vi "test_read-nmea-data2.vi"() -> ()   [LabVIEW 2019] (continued)
,86,148,25,33,59,218,30,1*43\n\t\n15:09:04.70\tF9P\t$GBGSV,2,1,05,08,,,28,10,,,07,11,51,130,29,14,86,148,31,3*7F\n\t\n15:09:04.72\tF9P\t$GBGSV,2,2,05,33,59,218,,3*46\n\t\n15:09:04.74\tF9P\t$GNGLL,3723.60830,N,12656.91746,E,060906.00,A,A*7D\n\t\n15:09:04.76\tF9P\t\t\n15:09:04.78\tF9P\t\t\n15:09:04.80\tF9P\t\t\n15:09:04.82\tF9P\t\t\n15:09:04.84\tF9P\t\t\n15:09:04.86\tF9P\t\t\n15:09:04.88\tF9P\t\t\n15:09:04.90\tF9P\t\t\n15:09:04.92\tF9P\t\t\n15:09:04.94\tF9P\t\t\n15:09:04.96\tF9P\t\t\n15:09:04.98\tF9P\t\t\n15:09:05.00\tF9P\t\t\n15:09:05.02\tF9P\t\t\n15:09:05.04\tF9P\t\t\n15:09:05.06\tF9P\t\t\n15:09:05.08\tF9P\t\t\n15:09:05.10\tF9P\t\t\n15:09:05.12\tF9P\t\t\n15:09:05.14\tF9P\t\t\n15:09:05.16\tF9P\t\t\n15:09:05.18\tF9P\t\t\n15:09:05.20\tF9P\t\t\n15:09:05.22\tF9P\t\t\n15:09:05.24\tF9P\t\t\n15:09:05.26\tF9P\t$GNRMC,060907.00,A,3723.60831,N,12656.91695,E,1.891,293.46,250720,,,A,V*06\n\t\n15:09:05.28\tF9P\t$GNVTG,293.46,T,,M,1.891,N,3.502,K,A*2C\n\t\n15:09:05.30\tF9P\t$GNGGA,060907.00,3723.60831,N,12656.91695,E,1,12,0.72,59.0,M,18.5,M,,*71\n\t\n15:09:05.32\tF9P\t$GNGSA,A,3,12,06,19,05,17,09,04,02,,,,,1.25,0.72,1.02,1*00\n\t\n15:09:05.34\tF9P\t$GNGSA,A,3,70,85,71,84,,,,,,,,,1.25,0.72,1.02,2*02\n\t\n15:09:05.36\tF9P\t$GNGSA,A,3,36,19,11,04,09,12,,,,,,,1.25,0.72,1.02,3*00\n\t\n15:09:05.38\tF9P\t$GNGSA,A,3,14,11,33,,,,,,,,,,1.25,0.72,1.02,4*01\n\t\n15:09:05.40\tF9P\t$GPGSV,3,1,09,02,54,318,26,04,19,044,26,05,36,246,25,06,65,046,28,1*60\n\t\n15:09:05.42\tF9P\t$GPGSV,3,2,09,09,45,076,35,12,24,278,29,17,35,153,24,19,54,156,24,1*6C\n\t\n15:09:05.44\tF9P\t$GPGSV,3,3,09,25,12,308,,1*52\n\t\n15:09:05.46\tF9P\t$GPGSV,3,1,09,02,54,318,,04,19,044,20,05,36,246,17,06,65,046,23,6*6F\n\t\n15:09:05.48\tF9P\t$GPGSV,3,2,09,09,45,076,20,12,24,278,22,17,35,153,,19,54,156,,6*64\n\t\n15:09:05.50\tF9P\t$GPGSV,3,3,09,25,12,308,,6*55\n\t\n15:09:05.52\tF9P\t$GLGSV,2,1,08,69,13,031,,70,73,042,21,71,50,204,27,72,03,209,,1*77\n\t\n15:09:05.54\tF9P\t$GLGSV,2,2,08,77,01,327,,84,21,121,10,85,70,063,25,86,35,329,,1*73\n\t\n15:09:05.56\tF9P\t$GLGSV,2,1,08,69,13,031,,70,73,042,,71,50,204,22,72,03,209,,3*73\n\t\n15:09:05.58\tF9P\t$GLGSV,2,2,08,77,01,327,,84,21,121,18,85,70,063,23,86,35,329,,3*7F\n\t\n15:09:05.60\tF9P\t$GAGSV,2,1,08,02,09,298,10,04,65,120,25,09,30,193,24,11,70,356,30,7*71\n\t\n15:09:05.62\tF9P\t$GAGSV,2,2,08,12,41,101,25,19,27,046,24,25,10,250,,36,25,307,20,7*76\n\t\n15:09:05.64\tF9P\t$GAGSV,2,1,08,02,09,298,,04,65,120,33,09,30,193,,11,70,356,27,2*72\n\t\n15:09:05.66\tF9P\t$GAGSV,2,2,08,12,41,101,20,19,27,046,19,25,10,250,,36,25,307,14,2*7F\n\t\n15:09:05.68\tF9P\t$GBGSV,1,1,03,11,51,130,26,14,86,148,25,33,59,218,29,1*4A\n\t\n15:09:05.70\tF9P\t$GBGSV,2,1,05,08,,,29,10,,,07,11,51,130,27,14,86,148,31,3*70\n\t\n15:09:05.72\tF9P\t$GBGSV,2,2,05,33,59,218,,3*46\n\t\n15:09:05.74\tF9P\t$GNGLL,3723.60831,N,12656.91695,E,060907.00,A,A*72\n\t\n15:09:05.76\tF9P\t\t\n15:09:05.78\tF9P\t\t\n15:09:05.80\tF9P\t\t\n15:09:05.82\tF9P\t\t\n15:09:05.84\tF9P\t\t\n15:09:05.86\tF9P\t\t\n15:09:05.88\tF9P\t\t\n15:09:05.90\tF9P\t\t\n15:09:05.92\tF9P\t\t\n15:09:05.94\tF9P\t\t\n15:09:05.96\tF9P\t\t\n15:09:05.98\tF9P\t\t\n15:09:06.00\tF9P\t\t\n15:09:06.02\tF9P\t\t\n15:09:06.04\tF9P\t\t\n15:09:06.06\tF9P\t\t\n15:09:06.08\tF9P\t\t\n15:09:06.10\tF9P\t\t\n15:09:06.12\tF9P\t\t\n15:09:06.14\tF9P\t\t\n15:09:06.16\tF9P\t\t\n15:09:06.18\tF9P\t\t\n15:09:06.20\tF9P\t\t\n15:09:06.22\tF9P\t\t\n15:09:06.24\tF9P\t\t\n15:09:06.26\tF9P\t$GNRMC,060908.00,A,3723.60810,N,12656.91634,E,2.095,270.86,250720,,,A,V*0F\n\t\n15:09:06.28\tF9P\t$GNVTG,270.86,T,,M,2.095,N,3.879,K,A*23\n\t\n15:09:06.30\tF9P\t$GNGGA,060908.00,3723.60810,N,12656.91634,E,1,12,0.68,59.0,M,18.5,M,,*7D\n\t\n15:09:06.32\tF9P\t$GNGSA,A,3,12,06,19,05,17,09,04,02,,,,,1.22,0.68,1.01,1*0F\n\t\n15:09:06.34\tF9P\t$GNGSA,A,3,70,85,71,84,,,,,,,,,1.22,0.68,1.01,2*0D\n\t\n15:09:06.36\tF9P\t$GNGSA,A,3,36,19,11,04,09,12,,,,,,,1.22,0.68,1.01,3*0F\n\t\n15:09:06.38\tF9P\t$GNGSA,A,3,14,11,33,,,,,,,,,,1.22,0.68,1.01,4*0E\n\t\n15:09:06.40\tF9P\t$GPGSV,3,1,09,02,54,318,25,04,19,044,26,05,36,246,28,06,65,046,29,1*6F\n\t\n15:09:06.42\tF9P\t$GPGSV,3,2,09,09,45,076,33,12,24,278,28,17,35,153,26,19,54,156,26,1*6B\n\t\n15:09:06.44\tF9P\t$GPGSV,3,3,09,25,12,308,,1*52\n\t\n15:09:06.46\tF9P\t$GPGSV,3,1,09,02,54,318,,04,19,044,20,05,36,246,19,06,65,046,25,6*67\n\t\n15:09:06.48\tF9P\t$GPGSV,3,2,09,09,45,076,21,12,24,278,21,17,35,153,,19,54,156,,6*66\n\t\n15:09:06.50\tF9P\t$GPGSV,3,3,09,25,12,308,,6*55\n\t\n15:09:06.52\tF9P\t$GLGSV,2,1,08,69,13,031,,70,73,042,18,71,50,204,27,72,03,209,,1*7D\n\t\n15:09:06.54\tF9P\t$GLGSV,2,2,08,77,01,327,,84,21,121,07,85,70,063,24,86,35,329,,1*74\n\t\n15:09:06.56\tF9P\t$GLGSV,2,1,08,69,13,031,21,70,73,042,,71,50,204,21,72,03,209,,3*73\n\t\n15:09:06.58\tF9P\t$GLGSV,2,2,08,77,01,327,,84,21,121,19,85,70,063,25,86,35,329,,3*78\n\t\n15:09:06.60\tF9P\t$GAGSV,2,1,08,02,09,298,07,04,65,120,24,09,30,193,24,11,70,356,24,7*73\n\t\n15:09:06.62\tF9P\t$GAGSV,2,2,08,12,41,101,23,19,27,046,20,25,10,250,,36,25,307,19,7*7E\n\t\n15:09:06.64\tF9P\t$GAGSV,2,1,08,02,09,298,,04,65,120,33,09,30,193,22,11,70,356,26,2*73\n\t\n15:09:06.66\tF9P\t$GAGSV,2,2,08,12,41,101,18,19,27,046,18,25,10,250,,36,25,307,20,2*72\n\t\n15:09:06.68\tF9P\t$GBGSV,1,1,03,11,51,130,25,14,86,148,30,33,59,218,29,1*4D\n\t\n15:09:06.70\tF9P\t$GBGSV,2,1,05,08,,,30,10,,,08,11,51,130,26,14,86,148,27,3*71\n\t\n15:09:06.72\tF9P\t$GBGSV,2,2,05,33,59,218,,3*46\n\t\n15:09:06.74\tF9P\t$GNGLL,3723.60810,N,12656.91634,E,060908.00,A,A*75\n\t\n15:09:06.76\tF9P\t\t\n15:09:06.78\tF9P\t\t\n15:09:06.80\tF9P\t\t\n15:09:06.82\tF9P\t\t\n15:09:06.84\tF9P\t\t\n15:09:06.86\tF9P\t\t\n15:09:06.88\tF9P\t\t\n15:09:06.90\tF9P\t\t\n15:09:06.92\tF9P\t\t\n15:09:06.94\tF9P\t\t\n15:09:06.96\tF9P\t\t\n15:09:06.98\tF9P\t\t\n15:09:07.00\tF9P\t\t\n15:09:07.02\tF9P\t\t\n15:09:07.04\tF9P\t\t\n15:09:07.06\tF9P\t\t\n15:09:07.08\tF9P\t\t\n15:09:07.10\tF9P\t\t\n15:09:07.12\tF9P\t\t\n15:09:07.14\tF9P\t\t\n15:09:07.16\tF9P\t\t\n15:09:07.18\tF9P\t\t\n15:09:07.20\tF9P\t\t\n15:09:07.22\tF9P\t\t\n15:09:07.24\tF9P\t\t\n15:09:07.26\tF9P\t$GNRMC,060909.00,A,3723.60783,N,12656.91558,E,2.757,256.79,250720,,,A,V*0F\n\t\n15:09:07.28\tF9P\t$GNVTG,256.79,T,,M,2.757,N,5.107,K,A*28\n\t\n15:09:07.30\tF9P\t$GNGGA,060909.00,3723.60783,N,12656.91558,E,1,12,0.69,59.0,M,18.5,M,,*71\n\t\n15:09:07.32\tF9P\t$GNGSA,A,3,12,06,19,05,17,09,04,02,,,,,1.25,0.69,1.04,1*0C\n\t\n15:09:07.34\tF9P\t$GNGSA,A,3,85,71,84,,,,,,,,,,1.25,0.69,1.04,2*09\n\t\n15:09:07.36\tF9P\t$GNGSA,A,3,36,19,11,04,09,12,,,,,,,1.25,0.69,1.04,3*0C\n\t\n15:09:07.38\tF9P\t$GNGSA,A,3,14,11,33,,,,,,,,,,1.25,0.69,1.04,4*0D\n\t\n15:09:07.40\tF9P\t$GPGSV,3,1,09,02,54,318,26,04,19,044,24,05,36,246,32,06,65,046,30,1*6D\n\t\n15:09:07.42\tF9P\t$GPGSV,3,2,09,09,45,075,35,12,24,278,21,17,35,153,24,19,54,156,31,1*63\n\t\n15:09:07.44\tF9P\t$GPGSV,3,3,09,25,12,308,,1*52\n\t\n15:09:07.46\tF9P\t$GPGSV,3,1,09,02,54,318,,04,19,044,20,05,36,246,19,06,65,046,26,6*64\n\t\n15:09:07.48\tF9P\t$GPGSV,3,2,09,09,45,075,21,12,24,278,21,17,35,153,,19,54,156,,6*65\n\t\n15:09:07.50\tF9P\t$GPGSV,3,3,09,25,12,308,,6*55\n\t\n15:09:07.52\tF9P\t$GLGSV,2,1,08,69,13,031,,70,73,042,,71,50,204,26,72,03,209,,1*75\n\t\n15:09:07.54\tF9P\t$GLGSV,2,2,08,77,01,327,,84,21,121,11,85,70,063,27,86,35,329,,1*70\n\t\n15:09:07.56\tF9P\t$GLGSV,2,1,08,69,13,031,20,70,73,042,,71,50,204,22,72,03,209,,3*71\n\t\n15:09:07.58\tF9P\t$GLGSV,2,2,08,77,01,327,,84,21,121,19,85,70,063,25,86,35,329,,3*78\n\t\n15:09:07.60\tF9P\t$GAGSV,2,1,08,02,09,298,06,04,65,120,26,09,30,193,24,11,70,356,25,7*71\n\t\n15:09:07.62\tF9P\t$GAGSV,2,2,08,12,41,101,22,19,27,046,18,25,10,250,,36,25,307,18,7*75\n\t\n15:09:07.64\tF9P\t$GAGSV,2,1,08,02,09,298,,04,65,120,33,09,30,193,21,11,70,356,23,2*75\n\t\n15:09:07.66\tF9P\t$GAGSV,2,2,08,12,41,101,18,19,27,046,17,25,10,250,,36,25,307,21,2*7C\n\t\n15:09:07.68\tF9P\t$GBGSV,1,1,03,11,51,130,23,14,86,148,24,33,59,218,28,1*4F\n\t\n15:09:07.70\tF9P\t$GBGSV,1,1,04,08,,,24,11,51,130,24,14,86,148,27,33,59,218,,3*4A\n\t\n15:09:07.72\tF9P\t$GNGLL,3723.60783,N,12656.91558,E,060909.00,A,A*78\n\t\n15:09:07.74\tF9P\t\t\n15:09:07.76\tF9P\t\t\n15:09:07.78\tF9P\t\t\n15:09:07.80\tF9P\t\t\n15:09:07.82\tF9P\t\t\n15:09:07.84\tF9P\t\t\n15:09:07.86\tF9P\t\t\n15:09:07.88\tF9P\t\t\n15:09:07.90\tF9P\t\t\n15:09:07.92\tF9P\t\t\n15:09:07.94\tF9P\t\t\n15:09:07.96\tF9P\t\t\n15:09:07.98\tF9P\t\t\n15:09:08.00\tF9P\t\t\n15:09:08.02\tF9P\t\t\n15:09:08.04\tF9P\t\t\n15:09:08.06\tF9P\t\t\n15:09:08.08\tF9P\t\t\n15:09:08.10\tF9P\t\t\n15:09:08.12\tF9P\t\t\n15:09:08.14\tF9P\t\t\n15:09:08.16\tF9P\t\t\n15:09:08.18\tF9P\t\t\n15:09:08.20\tF9P\t\t\n15:09:08.22\tF9P\t\t\n15:09:08.24\tF9P\t\t\n15:09:08.26\tF9P\t$GNRMC,060910.00,A,3723.60766,N,12656.91507,E,1.541,,250720,,,A,V*11\n\t\n15:09:08.28\tF9P\t$GNVTG,,T,,M,1.541,N,2.853,K,A*30\n\t\n15:09:08.30\tF9P\t$GNGGA,060910.00,3723.60766,N,12656.91507,E,1,12,0.69,59.3,M,18.5,M,,*7B\n\t\n15:09:08.32\tF9P\t$GNGSA,A,3,12,06,19,05,17,09,04,02,,,,,1.25,0.69,1.04,1*0C\n\t\n15:09:08.34\tF9P\t$GNGSA,A,3,85,71,84,,,,,,,,,,1.25,0.69,1.04,2*09\n\t\n15:09:08.36\tF9P\t$GNGSA,A,3,36,19,11,04,09,12,,,,,,,1.25,0.69,1.04,3*0C\n\t\n15:09:08.38\tF9P\t$GNGSA,A,3,14,11,33,,,,,,,,,,1.25,0.69,1.04,4*0D\n\t\n15:09:08.40\tF9P\t$GPGSV,3,1,09,02,54,318,24,04,19,044,23,05,36,246,27,06,65,046,30,1*6C\n\t\n15:09:08.42\tF9P\t$GPGSV,3,2,09,09,45,075,27,12,24,278,23,17,35,153,25,19,54,156,24,1*67\n\t\n15:09:08.44\tF9P\t$GPGSV,3,3,09,25,12,308,,1*52\n\t\n15:09:08.46\tF9P\t$GPGSV,3,1,09,02,54,318,,04,19,044,19,05,36,246,18,06,65,046,27,6*6E\n\t\n15:09:08.48\tF9P\t$GPGSV,3,2,09,09,45,075,23,12,24,278,19,17,35,153,22,19,54,156,,6*6C\n\t\n15:09:08.50\tF9P\t$GPGSV,3,3,09,25,12,308,,6*55\n\t\n15:09:08.52\tF9P\t$GLGSV,2,1,08,69,13,031,,70,73,042,,71,50,204,26,72,03,209,,1*75\n\t\n15:09:08.54\tF9P\t$GLGSV,2,2,08,77,01,327,,84,21,121,10,85,70,063,26,86,35,329,,1*70\n\t\n15:09:08.56\tF9P\t$GLGSV,2,1,08,69,13,031,19,70,73,042,,71,50,204,21,72,03,209,,3*78\n\t\n15:09:08.58\tF9P\t$GLGSV,2,2,08,77,01,327,,84,21,121,19,85,70,063,25,86,35,329,,3*78\n\t\n15:09:08.60\tF9P\t$GAGSV,2,1,08,02,09,298,09,04,65,120,25,09,30,193,27,11,70,356,26,7*7D\n\t\n15:09:08.62\tF9P\t$GAGSV,2,2,08,12,41,101,29,19,27,046,17,25,10,250,,36,25,307,18,7*71\n\t\n15:09:08.64\tF9P\t$GAGSV,2,1,08,02,09,298,,04,65,120,33,09,30,193,20,11,70,356,23,2*74\n\t\n15:09:08.66\tF9P\t$GAGSV,2,2,08,12,41,101,17,19,27,046,16,25,10,250,,36,25,307,23,2*70\n\t\n15:09:08.68\tF9P\t$GBGSV,1,1,03,11,51,130,22,14,86,148,24,33,59,218,28,1*4E\n\t\n15:09:08.70\tF9P\t$GBGSV,1,1,04,08,,,22,11,51,130,21,14,86,148,27,33,59,218,,3*49\n\t\n15:09:08.72\tF9P\t$GNGLL,3723.60766,N,12656.91507,E,060910.00,A,A*71\n\t\n15:09:08.74\tF9P\t\t\n15:09:08.76\tF9P\t\t\n15:09:08.78\tF9P\t\t\n15:09:08.80\tF9P\t\t\n15:09:08.82\tF9P\t\t\n15:09:08.84\tF9P\t\t\n15:09:08.86\tF9P\t\t\n15:09:08.88\tF9P\t\t\n15:09:08.90\tF9P\t\t\n15:09:08.92\tF9P\t\t\n15:09:08.94\tF9P\t\t\n15:09:08.96\tF9P\t\t\n15:09:08.98\tF9P\t\t\n15:09:09.00\tF9P\t\t\n15:09:09.02\tF9P\t\t\n15:09:09.04\tF9P\t\t\n15:09:09.06\tF9P\t\t\n15:09:09.08\tF9P\t\t\n15:09:09.10\tF9P\t\t\n15:09:09.12\tF9P\t\t\n15:09:09.14\tF9P\t\t\n15:09:09.16\tF9P\t\t\n15:09:09.18\tF9P\t\t\n15:09:09.20\tF9P\t\t\n15:09:09.22\tF9P\t\t\n15:09:09.24\tF9P\t\t\n15:09:09.26\tF9P\t$GNRMC,060911.00,A,3723.60762,N,12656.91440,E,2.158,259.99,250720,,,A,V*09\n\t\n15:09:09.28\tF9P\t$GNVTG,259.99,T,,M,2.158,N,3.997,K,A*27\n\t\n15:09:09.30\tF9P\t$GNGGA,060911.00,3723.60762,N,12656.91440,E,1,12,0.73,59.5,M,18.5,M,,*71\n\t\n15:09:09.32\tF9P\t$GNGSA,A,3,12,06,19,05,17,09,04,02,,,,,1.28,0.73,1.05,1*0B\n\t\n15:09:09.34\tF9P\t$GNGSA,A,3,85,71,84,,,,,,,,,,1.28,0.73,1.05,2*0E\n\t\n15:09:09.36\tF9P\t$GNGSA,A,3,36,19,11,04,09,12,,,,,,,1.28,0.73,1.05,3*0B\n\t\n15:09:09.38\tF9P\t$GNGSA,A,3,14,11,33,,,,,,,,,,1.28,0.73,1.05,4*0A\n\t\n15:09:09.40\tF9P\t$GPGSV,3,1,09,02,54,318,24,04,19,044,22,05,36,246,19,06,65,046,30,1*60\n\t\n15:09:09.42\tF9P\t$GPGSV,3,2,09,09,45,075,29,12,24,278,31,17,35,153,25,19,54,156,23,1*6D\n\t\n15:09:09.44\tF9P\t$GPGSV,3,3,09,25,12,308,,1*52\n\t\n15:09:09.46\tF9P\t$GPGSV,3,1,09,02,54,318,,04,19,044,17,05,36,246,17,06,65,046,28,6*60\n\t\n15:09:09.48\tF9P\t$GPGSV,3,2,09,09,45,075,24,12,24,278,19,17,35,153,19,19,54,156,,6*63\n\t\n15:09:09.50\tF9P\t$GPGSV,3,3,09,25,12,308,,6*55\n\t\n15:09:09.52\tF9P\t$GLGSV,2,1,08,69,13,031,,70,73,042,,71,50,204,27,72,03,209,,1*74\n\t\n15:09:09.54\tF9P\t$GLGSV,2,2,08,77,01,327,,84,21,121,11,85,70,063,25,86,35,329,,1*72\n\t\n15:09:09.56\tF9P\t$GLGSV,2,1,08,69,13,031,20,70,73,042,,71,50,204,23,72,03,209,,3*70\n\t\n15:09:09.58\tF9P\t$GLGSV,2,2,08,77,01,327,,84,21,121,18,85,70,063,23,86,35,329,,3*7F\n\t\n15:09:09.60\tF9P\t$GAGSV,2,1,08,02,09,298,09,04,65,120,24,09,30,193,26,11,70,356,26,7*7D\n\t\n15:09:09.62\tF9P\t$GAGSV,2,2,08,12,41,101,22,19,27,046,15,25,10,250,,36,25,307,17,7*77\n\t\n15:09:09.64\tF9P\t$GAGSV,2,1,08,02,09,298,,04,65,120,33,09,30,193,22,11,70,356,23,2*76\n\t\n15:09:09.66\tF9P\t$GAGSV,2,2,08,12,41,101,18,19,27,046,14,25,10,250,,36,25,307,24,2*7A\n\t\n15:09:09.68\tF9P\t$GBGSV,1,1,03,11,51,130,21,14,86,148,25,33,59,218,27,1*43\n\t\n15:09:09.70\tF9P\t$GBGSV,1,1,04,08,,,22,11,51,130,20,14,86,148,27,33,59,218,,3*48\n\t\n15:09:09.72\tF9P\t$GNGLL,3723.60762,N,12656.91440,E,060911.00,A,A*76\n\t\n15:09:09.74\tF9P\t\t\n15:09:09.76\tF9P\t\t\n15:09:09.78\tF9P\t\t\n15:09:09.80\tF9P\t\t\n15:09:09.82\tF9P\t\t\n15:09:09.84\tF9P\t\t\n15:09:09.86\tF9P\t\t\n15:09:09.88\tF9P\t\t\n15:09:09.90\tF9P\t\t\n15:09:09.92\tF9P\t\t\n15:09:09.94\tF9P\t\t\n15:09:09.96\tF9P\t\t\n15:09:09.98\tF9P\t\t\n15:09:10.00\tF9P\t\t\n15:09:10.02\tF9P\t\t\n15:09:10.04\tF9P\t\t\n15:09:10.06\tF9P\t\t\n15:09:10.08\tF9P\t\t\n15:09:10.10\tF9P\t\t\n15:09:10.12\tF9P\t\t\n15:09:10.14\tF9P\t\t\n15:09:10.16\tF9P\t\t\n15:09:10.18\tF9P\t\t\n15:09:10.20\tF9P\t\t\n15:09:10.22\tF9P\t\t\n15:09:10.24\tF9P\t\t\n15:09:10.26\tF9P\t$GNRMC,060912.00,A,3723.60754,N,12656.91377,E,1.994,258.61,250720,,,A,V*01\n\t\n15:09:10.28\tF9P\t$GNVTG,258.61,T,,M,1.994,N,3.693,K,A*21\n\t\n15:09:10.30\tF9P\t$GNGGA,060912.00,3723.60754,N,12656.91377,E,1,12,0.73,59.9,M,18.5,M,,*78\n\t\n15:09:10.32\tF9P\t$GNGSA,A,3,12,06,19,05,17,09,04,02,,,,,1.28,0.73,1.05,1*0B\n\t\n15:09:10.34\tF9P\t$GNGSA,A,3,85,71,84,,,,,,,,,,1.28,0.73,1.05,2*0E\n\t\n15:09:10.36\tF9P\t$GNGSA,A,3,36,19,11,04,09,12,,,,,,,1.28,0.73,1.05,3*0B\n\t\n15:09:10.38\tF9P\t$GNGSA,A,3,14,11,33,,,,,,,,,,1.28,0.73,1.05,4*0A\n\t\n15:09:10.40\tF9P\t$GPGSV,3,1,09,02,54,318,23,04,19,044,20,05,36,246,29,06,65,046,28,1*6F\n\t\n15:09:10.42\tF9P\t$GPGSV,3,2,09,09,45,075,33,12,24,278,24,17,35,153,24,19,54,156,23,1*63\n\t\n15:09:10.44\tF9P\t$GPGSV,3,3,09,25,12,308,,1*52\n\t\n15:09:10.46\tF9P\t$GPGSV,3,1,09,02,54,318,,04,19,044,14,05,36,246,16,06,65,046,28,6*62\n\t\n15:09:10.48\tF9P\t$GPGSV,3,2,09,09,45,075,24,12,24,278,17,17,35,153,17,19,54,156,,6*63\n\t\n15:09:10.50\tF9P\t$GPGSV,3,3,09,25,12,308,,6*55\n\t\n15:09:10.52\tF9P\t$GLGSV,2,1,08,69,13,031,,70,73,042,,71,50,204,32,72,03,209,,1*70\n\t\n15:09:10.54\tF9P\t$GLGSV,2,2,08,77,01,327,,84,21,121,09,85,70,063,25,86,35,329,,1*7B\n\t\n15:09:10.56\tF9P\t$GLGSV,2,1,08,69,13,031,20,70,73,042,,71,50,204,25,72,03,209,,3*76\n\t\n15:09:10.58\tF9P\t$GLGSV,2,2,08,77,01,327,,84,21,121,18,85,70,063,22,86,35,329,,3*7E\n\t\n15:09:10.60\tF9P\t$GAGSV,2,1,08,02,09,298,08,04,65,120,25,09,30,193,25,11,70,356,26,7*7E\n\t\n15:09:10.62\tF9P\t$GAGSV,2,2,08,12,41,101,23,19,27,046,13,25,10,250,,36,25,307,18,7*7F\n\t\n15:09:10.64\tF9P\t$GAGSV,2,1,08,02,09,298,,04,65,120,32,09,30,193,22,11,70,356,25,2*71\n\t\n15:09:10.66\tF9P\t$GAGSV,2,2,08,12,41,101,18,19,27,046,13,25,10,250,,36,25,307,23,2*7A\n\t\n15:09:10.68\tF9P\t$GBGSV,1,1,03,11,51,130,22,14,86,148,26,33,59,218,27,1*43\n\t\n15:09:10.70\tF9P\t$GBGSV,1,1,04,08,,,23,11,51,130,21,14,86,148,20,33,59,218,,3*4F\n\t\n15:09:10.72\tF9P\t$GNGLL,3723.60754,N,12656.91377,E,060912.00,A,A*73\n\t\n15:09:10.74\tF9P\t\t\n15:09:10.76\tF9P\t\t\n15:09:10.78\tF9P\t\t\n15:09:10.80\tF9P\t\t\n15:09:10.82\tF9P\t\t\n15:09:10.84\tF9P\t\t\n15:09:10.86\tF9P\t\t\n15:09:10.88\tF9P\t\t\n15:09:10.90\tF9P\t\t\n15:09:10.92\tF9P\t\t\n15:09:10.94\tF9P\t\t\n15:09:10.96\tF9P\t\t\n15:09:10.98\tF9P\t\t\n15:09:11.00\tF9P\t\t\n15:09:11.02\tF9P\t\t\n15:09:11.04\tF9P\t\t\n15:09:11.06\tF9P\t\t\n15:09:11.08\tF9P\t\t\n15:09:11.10\tF9P\t\t\n15:09:11.12\tF9P\t\t\n15:09:11.14\tF9P\t\t\n15:09:11.16\tF9P\t\t\n15:09:11.18\tF9P\t\t\n15:09:11.20\tF9P\t\t\n15:09:11.22\tF9P\t\t\n15:09:11.24\tF9P\t\t\n15:09:11.26\tF9P\t$GNRMC,060913.00,A,3723.60728,N,12656.91303,E,2.755,249.40,250720,,,A,V*0B\n\t\n15:09:11.29\tF9P\t$GNVTG,249.40,T,,M,2.755,N,5.102,K,A*2B\n\t\n15:09:11.31\tF9P\t$GNGGA,060913.00,3723.60728,N,12656.91303,E,1,12,0.73,59.1,M,18.5,M,,*79\n\t\n15:09:11.33\tF9P\t$GNGSA,A,3,12,06,19,05,17,09,04,02,,,,,1.28,0.73,1.05,1*0B\n\t\n15:09:11.35\tF9P\t$GNGSA,A,3,85,71,84,,,,,,,,,,1.28,0.73,1.05,2*0E\n\t\n15:09:11.37\tF9P\t$GNGSA,A,3,36,19,11,04,09,12,,,,,,,1.28,0.73,1.05,3*0B\n\t\n15:09:11.39\tF9P\t$GNGSA,A,3,14,11,33,,,,,,,,,,1.28,0.73,1.05,4*0A\n\t\n15:09:11.41\tF9P\t$GPGSV,3,1,09,02,54,318,23,04,19,044,19,05,36,246,28,06,65,046,28,1*64\n\t\n15:09:11.43\tF9P\t$GPGSV,3,2,09,09,45,075,34,12,24,278,25,17,35,153,23,19,54,156,23,1*62\n\t\n15:09:11.45\tF9P\t$GPGSV,3,3,09,25,12,308,,1*52\n\t\n15:09:11.47\tF9P\t$GPGSV,3,1,09,02,54,318,,04,19,044,16,05,36,246,16,06,65,046,27,6*6F\n\t\n15:09:11.49\tF9P\t$GPGSV,3,2,09,09,45,075,22,12,24,278,17,17,35,153,16,19,54,156,,6*64\n\t\n15:09:11.51\tF9P\t$GPGSV,3,3,09,25,12,308,,6*55\n\t\n15:09:11.53\tF9P\t$GLGSV,2,1,08,69,13,031,,70,73,042,,71,50,204,26,72,03,209,,1*75\n\t\n15:09:11.55\tF9P\t$GLGSV,2,2,08,77,01,327,,84,21,121,09,85,70,063,26,86,35,329,,1*78\n\t\n15:09:11.57\tF9P\t$GLGSV,2,1,08,69,13,031,18,70,73,042,,71,50,204,24,72,03,209,,3*7C\n\t\n15:09:11.59\tF9P\t$GLGSV,2,2,08,77,01,327,,84,21,121,18,85,70,063,22,86,35,329,,3*7E\n\t\n15:09:11.61\tF9P\t$GAGSV,2,1,08,02,09,298,10,04,65,120,26,09,30,193,30,11,70,356,24,7*72\n\t\n15:09:11.63\tF9P\t$GAGSV,2,2,08,12,41,101,22,19,27,046,13,25,10,250,,36,25,307,17,7*71\n\t\n15:09:11.65\tF9P\t$GAGSV,2,1,08,02,09,298,,04,65,120,28,09,30,193,24,11,70,356,23,2*7A\n\t\n15:09:11.67\tF9P\t$GAGSV,2,2,08,12,41,101,17,19,27,046,09,25,10,250,,36,25,307,24,2*79\n\t\n15:09:11.69\tF9P\t$GBGSV,1,1,03,11,51,130,24,14,86,148,25,33,59,218,27,1*46\n\t\n15:09:11.71\tF9P\t$GBGSV,1,1,04,08,,,23,11,51,130,23,14,86,148,27,33,59,218,,3*4A\n\t\n15:09:11.73\tF9P\t$GNGLL,3723.60728,N,12656.91303,E,060913.00,A,A*7A\n\t\n15:09:11.75\tF9P\t\t\n15:09:11.77\tF9P\t\t\n15:09:11.79\tF9P\t\t\n15:09:11.81\tF9P\t\t\n15:09:11.83\tF9P\t\t\n15:09:11.85\tF9P\t\t\n15:09:11.87\tF9P\t\t\n15:09:11.89\tF9P\t\t\n15:09:11.91\tF9P\t\t\n15:09:11.93\tF9P\t\t\n15:09:11.95\tF9P\t\t\n15:09:11.97\tF9P\t\t\n15:09:11.99\tF9P\t\t\n15:09:12.01\tF9P\t\t\n15:09:12.03\tF9P\t\t\n15:09:12.05\tF9P\t\t\n15:09:12.07\tF9P\t\t\n15:09:12.09\tF9P\t\t\n15:09:12.11\tF9P\t\t\n15:09:12.13\tF9P\t\t\n15:09:12.15\tF9P\t\t\n15:09:12.17\tF9P\t\t\n15:09:12.19\tF9P\t\t\n15:09:12.21\tF9P\t\t\n15:09:12.23\tF9P\t\t\n15:09:12.25\tF9P\t$GNRMC,060914.00,A,3723.60695,N,12656.91212,E,2.899,243.18,250720,,,A,V*02\n\t\n15:09:12.27\tF9P\t$GNVTG,243.18,T,,M,2.899,N,5.370,K,A*24\n\t\n15:09:12.29\tF9P\t$GNGGA,060914.00,3723.60695,N,12656.91212,E,1,12,0.73,58.8,M,18.5,M,,*70\n\t\n15:09:12.31\tF9P\t$GNGSA,A,3,12,06,19,05,17,09,04,02,,,,,1.28,0.73,1.05,1*0B\n\t\n15:09:12.33\tF9P\t$GNGSA,A,3,85,71,84,,,,,,,,,,1.28,0.73,1.05,2*0E\n\t\n15:09:12.35\tF9P\t$GNGSA,A,3,36,19,11,04,09,12,,,,,,,1.28,0.73,1.05,3*0B\n\t\n15:09:12.37\tF9P\t$GNGSA,A,3,14,11,33,,,,,,,,,,1.28,0.73,1.05,4*0A\n\t\n15:09:12.39\tF9P\t$GPGSV,3,1,09,02,54,318,23,04,19,044,19,05,36,246,27,06,65,046,28,1*6B\n\t\n15:09:12.41\tF9P\t$GPGSV,3,2,09,09,45,075,29,12,24,278,25,17,35,153,24,19,54,156,30,1*6B\n\t\n15:09:12.43\tF9P\t$GPGSV,3,3,09,25,12,308,,1*52\n\t\n15:09:12.45\tF9P\t$GPGSV,3,1,09,02,54,318,,04,19,044,15,05,36,246,16,06,65,046,26,6*6D\n\t\n15:09:12.47\tF9P\t$GPGSV,3,2,09,09,45,075,21,12,24,278,17,17,35,153,17,19,54,156,,6*66\n\t\n15:09:12.49\tF9P\t$GPGSV,3,3,09,25,12,308,,6*55\n\t\n15:09:12.51\tF9P\t$GLGSV,2,1,08,69,13,031,,70,73,042,,71,50,204,26,72,03,209,,1*75\n
